vi "xdevice_sub.vi"() -> ()   [LabVIEW 2019]
panel:
  out "Device moved":bool
  in  "Wavelength":dbl=795.0
  out "Temperature":dbl
  out "Serial number":string
  out "Wavelength":dbl
  out "Angle":dbl
  out "Device detected":bool
  out "Error message":string
  in  "xphyspecLib.IXPhySpec":refnum<k7>
  # "Device status"
  # "Device information"
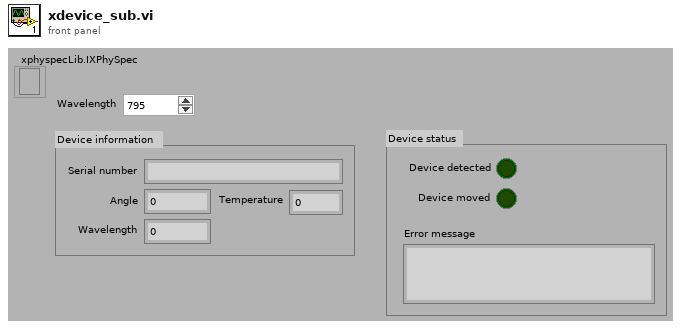
[diagram p1: front panel]
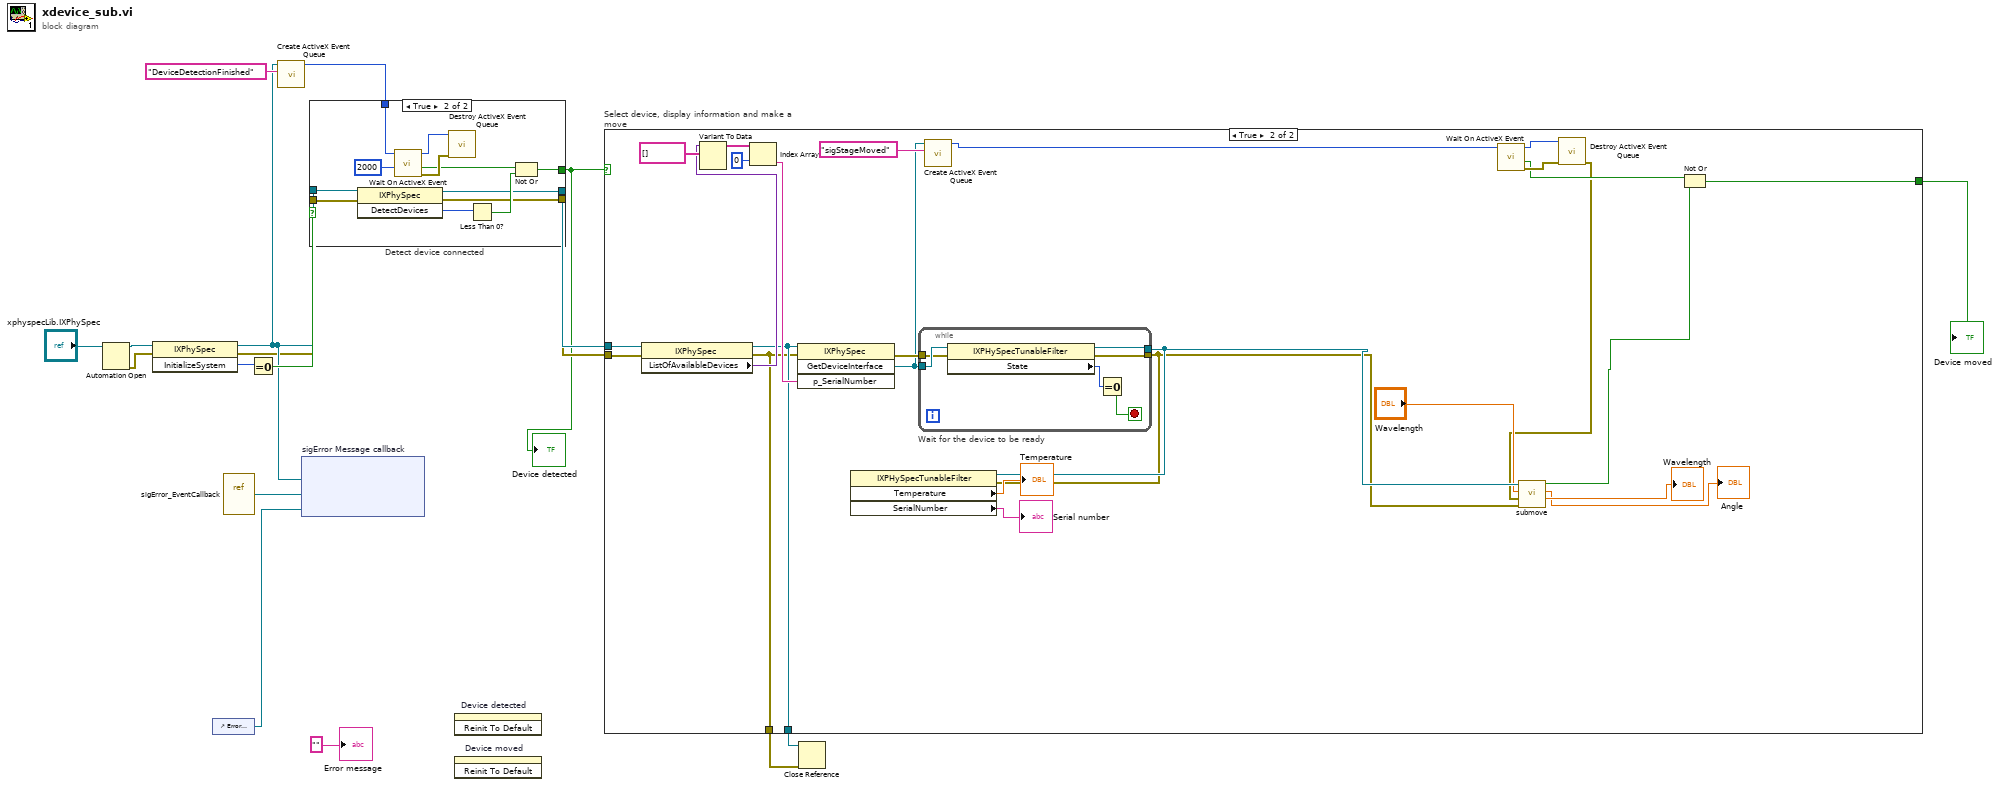
[diagram p0: block diagram]
diagram:
  n1 = Automation Open(Automation Refnum="xphyspecLib.IXPhySpec") -> (Automation Refnum=w17:refnum<k7>, error out=w16:errorcluster)  [unwired: 3 in]
  n2 = invoke class="IXPhySpec" method="InitializeSystem"(reference=w17, error in=w16) -> (reference out=w10:refnum<k7>, error out=w9:errorcluster, "InitializeSystem"=w15:i32)  [unwired: 1 in]
  n3 = control-ref of="Error message"() -> (w14:refnum<vi>)
  n4 = vi-ref "sigError_EventCallback.vi"() -> ("vi reference"=w13:refnum<vi>)
  n5 = Equal To 0?(x=w15) -> (x = 0?=w11:bool)
  n6 = call <vilib>:"Create ActiveX Event Queue.vi"("Event Name"="DeviceDetectionFinished", "Automation Refnum"=w10) -> ("Event Queue"=w8:i32)  [unwired: 4 in, 1 out]
  n7 = node "sigError Message callback"(w10, w13, w14) -> ()  [unwired: 2 in, 2 out]
  n8 = case "Detect device connected" shown="True" w11 {
    selector: w11 -> [w21 _]
    tunnel: w10 -> [w20 w33]
    tunnel: w9 -> [w19 w32]
    tunnel: w8 -> [_ w29]
    tunnel: [w20 w24] -> w7
    tunnel: [w19 w23] -> w6
    tunnel: [w21 w22] -> w5
    frame False {
    }
    frame True {
      n9 = invoke class="IXPhySpec" method="DetectDevices"(reference=w33, error in=w32) -> (reference out=w24:refnum<k7>, error out=w23:errorcluster, "DetectDevices"=w27:i32)  [unwired: 1 in]
      n10 = call <vilib>:"Wait On ActiveX Event.vi"("ms Timeout (-1)"=2000, "Event Queue"=w29) -> ("error out"=w28:errorcluster, "Timed Out"=w26:bool, "Event Queue Out"=w30:i32)  [unwired: 2 in, 1 out]
      n11 = call <vilib>:"Destroy ActiveX Event Queue.vi"("error in (no error)"=w28, "Event Queue"=w30) -> ()  [unwired: 5 in, 1 out]
      n12 = Less Than 0?(x=w27) -> (x < 0?=w25:bool)
      n13 = Not Or(1:w25, 2:w26) -> (0:w22:bool)
    }
  }
  "Device detected" <- w5
  n14 = invoke on="Device detected" class="Bool (strict)" method="Reinit To Default"() -> ()  [unwired: 3 in, 3 out]
  n15 = invoke on="Device moved" class="Bool (strict)" method="Reinit To Default"() -> ()  [unwired: 3 in, 3 out]
  n16 = case "Select device, display information and make a move" shown="True" w5 {
    selector: w5 -> [w36 _]
    tunnel: w7 -> [w35 w57]
    tunnel: w6 -> [w34 w56]
    tunnel: [w36 w48] -> w4
    tunnel: [w35 w47] -> w3
    tunnel: [w34 w46] -> w2
    frame False {
    }
    frame True {
      n17 = property class="IXPhySpec"(reference=w57, error in=w56) -> (reference out=w47:refnum<k7>, error out=w46:errorcluster, "ListOfAvailableDevices"=w59:variant)
      n18 = Variant To Data(type=string[] [], Variant=w59) -> (data=w61:string[])  [unwired: 1 in, 1 out]
      n19 = Index Array(array=w61, index=0) -> (element=w58:string)
      n20 = invoke class="IXPhySpec" method="GetDeviceInterface"(reference=w47, error in=w46, "p_SerialNumber"=w58) -> (error out=w55:errorcluster, "GetDeviceInterface"=w53:refnum<k7>)  [unwired: 1 in, 2 out]
      n21 = while "Wait for the device to be ready" {
        tunnel: [w66] -> w42
        tunnel: w53 -> [w65]
        tunnel: w55 -> [w64]
        tunnel: [w63] -> w43
        stop <- w67 stop-if-true
        n22 = property class="IXPHySpecTunableFilter"(reference=w65, error in=w64) -> (reference out=w63:refnum<k7>, error out=w66:errorcluster, "State"=w68:u32)
        n23 = Equal To 0?(x=w68) -> (x = 0?=w67:bool)
      }
      n24 = property class="IXPHySpecTunableFilter"(reference=w43, error in=w42) -> ("Temperature"=→"Temperature":dbl, "SerialNumber"=→"Serial number":string)  [unwired: 2 out]
      n25 = call <vilib>:"Create ActiveX Event Queue.vi"("Event Name"="sigStageMoved", "Automation Refnum"=w53) -> ("Event Queue"=w52:i32)  [unwired: 4 in, 1 out]
      n26 = call <vilib>:"Wait On ActiveX Event.vi"("Event Queue"=w52) -> ("error out"=w50:errorcluster, "Timed Out"=w49:bool, "Event Queue Out"=w51:i32)  [unwired: 3 in, 1 out]
      n27 = call <vilib>:"Destroy ActiveX Event Queue.vi"("error in (no error)"=w50, "Event Queue"=w51) -> ("error out"=w37:errorcluster)  [unwired: 5 in]
      n28 = call "submove.vi"("error in (no error)"=w42, "error in (no error) 2"=w37, "Wavelength"="Wavelength", "reference"=w43) -> ("Wavelength 2"=→"Wavelength":dbl, "Angle"=→"Angle":dbl, "x < 0?"=w40:bool)  [unwired: 5 in]
      n29 = Not Or(1:w40, 2:w49) -> (0:w48:bool)
    }
  }
  "Device moved" <- w4
  n30 = Close Reference(reference=w3, error in (no error)=w2) -> ()  [unwired: 1 out]
  "Error message" <- "" ("Error message")
